vi "WPI_DashboardUnpack DB data.vi"(11 "DB Packed Data":T2) -> (3 "output values":T1)   [LabVIEW 2017]
uses:
  <vilib>/Rock Robotics/WPI/Dashboard/WPI_DashboardDStoPCPacketTypeDef.ctl
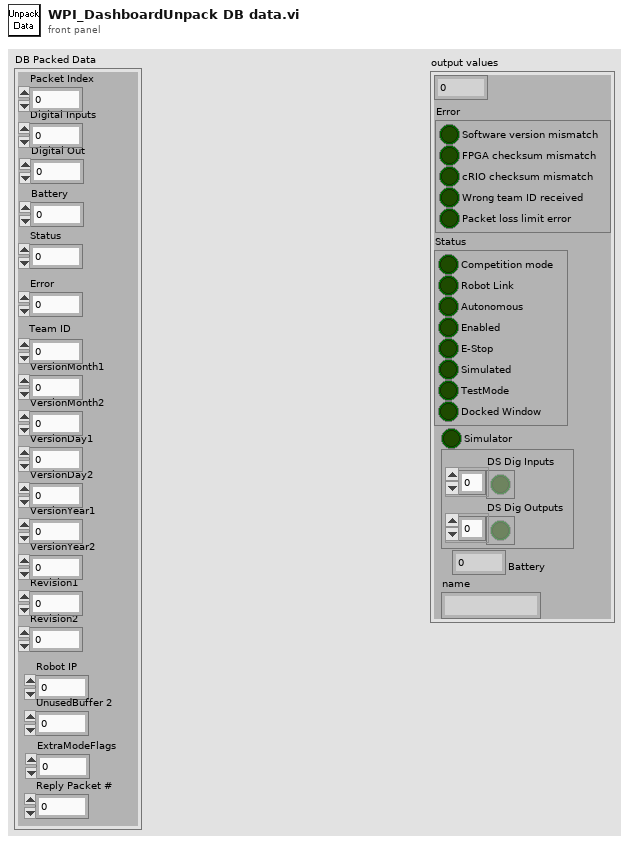
[diagram p1: front panel]
types:
  T1 = cluster{u16, "Error":cluster{"Software version mismatch":bool, "FPGA checksum mismatch":bool, "cRIO checksum mismatch":bool, "Wrong team ID received":bool, "Packet loss limit error":bool}, "Status":cluster{"Competition mode":bool, "Robot Link":bool, "Autonomous":bool, "Enabled":bool, "E-Stop":bool, "Simulated":bool, "TestMode":bool, "Docked Window":bool}, "Simulator":bool, cluster{"DS Dig Inputs":bool[], "DS Dig Outputs":bool[]}, "Battery":sgl, "name":string}
  T2 = typedef "WPI_DashboardDStoPCPacketTypeDef.ctl" = cluster{"Packet Index":u16, "Digital Inputs":u8, "Digital Out":u8, "Battery":u16, "Status":u8, "Error":u8, "Team ID":u16, "VersionMonth1":u8, "VersionMonth2":u8, "VersionDay1":u8, "VersionDay2":u8, "VersionYear1":u8, "VersionYear2":u8, "Revision1":u8, "Revision2":u8, "Robot IP":u32, "UnusedBuffer 2":u8, "ExtraModeFlags":u8, "Reply Packet #":u16}
  T3 = cluster{"Boolean array[0]":bool, "Boolean array[1]":bool, "Boolean array[2]":bool, "Boolean array[3]":bool, "Boolean array[4]":bool, "Boolean array[5]":bool, "Boolean array[6]":bool, "Boolean array[7]":bool}
  T4 = cluster{"Boolean array":bool[], "Boolean array":bool[]}
  T5 = cluster{"Boolean array[0]":bool, "Boolean array[1]":bool, "Boolean array[4]":bool, "Boolean array[5]":bool, bool, bool, bool, bool}
  T6 = cluster{u16, cluster{bool, bool, bool, bool, bool}, cluster{"Boolean array[0]":bool, "Boolean array[1]":bool, "Boolean array[4]":bool, "Boolean array[5]":bool, bool, bool, bool, bool}, bool, cluster{"Boolean array":bool[], "Boolean array":bool[]}, sgl, "name":string}
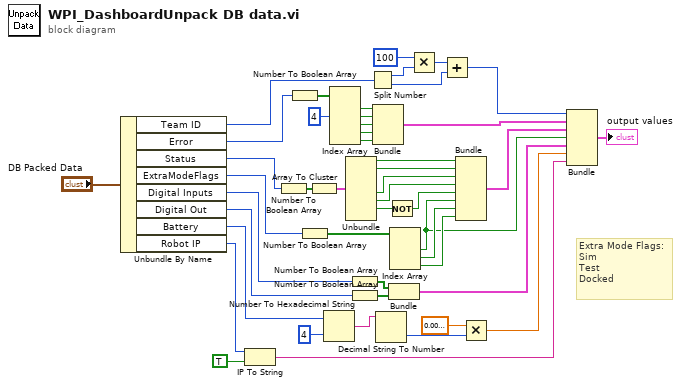
[diagram p0: block diagram]
diagram:
  # "Extra Mode Flags:\nSim\nTest\nDocked"
  n1 = Unbundle By Name("DB Packed Data") -> ("Team ID"=w42:u16, "Error"=w37:u8, "Status"=w22:u8, "ExtraModeFlags"=w21:u8, "Digital Inputs"=w17:u8, "Digital Out"=w18:u8, "Battery"=w12:u16, "Robot IP"=w10:u32)
  n2 = IP To String(1:TRUE ("dot notation? (F)"), 2:w10) -> (0:w2:string)
  n3 = Number To Boolean Array(number=w22) -> (Boolean array=w23:bool[])
  n4 = Number To Boolean Array(number=w37) -> (Boolean array=w38:bool[])
  n5 = Number To Boolean Array(number=w21) -> (Boolean array=w31:bool[])
  n6 = Array To Cluster(array=w23) -> (cluster=w24:T3)
  n7 = Number To Hexadecimal String(1:i16 4 ("width (-)"), 2:w12) -> (0:w14:string)
  n8 = Index Array(array=w38, index #2=4 ("index")) -> (element #1=w41:bool, element #2=w40:bool, element #3=w36:bool, element #4=w35:bool, element #5=w34:bool)  [unwired: 4 in]
  n9 = Unbundle(w24) -> ("Boolean array[0]"=w25:bool, "Boolean array[1]"=w26:bool, "Boolean array[4]"=w27:bool, "Boolean array[5]"=w28:bool, "Boolean array[6]"=w29:bool)  [unwired: 3 out]
  n10 = Number To Boolean Array(number=w17) -> (Boolean array=w20:bool[])
  n11 = Number To Boolean Array(number=w18) -> (Boolean array=w19:bool[])
  n12 = Split Number(x=w42) -> (hi(x)=w43:u8, lo(x)=w46:u8)
  n13 = Bundle(w41, w40, w36, w35, w34) -> (w7:cluster{bool, bool, bool, bool, bool})  [unwired: 1 out]
  n14 = Decimal String To Number(string=w14) -> (number=w16:i32)  [unwired: 3 out]
  n15 = Not(x=w29) -> (.not. x?=w30:bool)
  n16 = Bundle("Boolean array"=w20, "Boolean array"=w19) -> (w4:T4)  [unwired: 1 out]
  n17 = Index Array(array=w31) -> (element #1=w5:bool, element #2=w32:bool, element #3=w33:bool)  [unwired: 3 in]
  n18 = Multiply(x=u16 100, y=w43) -> (x*y=w45:u16)
  n19 = Add(x=w45, y=w46) -> (x+y=w8:u16)
  n20 = Bundle("Boolean array[0]"=w25, "Boolean array[1]"=w26, "Boolean array[4]"=w27, "Boolean array[5]"=w28, w30, w5, w32, w33) -> (w6:T5)  [unwired: 1 out]
  n21 = Multiply(x=sgl 0.01, y=w16) -> (x*y=w3:sgl)
  n22 = Bundle(w8, w7, w6, w5, w4, w3, "name"=w2) -> (→"output values":T6)  [unwired: 1 out]
